vi "Set Next Parameter.vi"(8 "error in (no error)":errorcluster, 10 "first?":bool, 11 "ExperimentService in":refnum<class "ExperimentService.lvclass">) -> (0 "error out":errorcluster, 3 "ExperimentService out":refnum<class "ExperimentService.lvclass">)   [LabVIEW 2014, in "ExperimentService.lvclass"]
uses:
  ExperimentService.lvclass
  ExperimentService.lvclass/ExperimentService.ctl
  Interfaces/Observable Actor/Observable Actor.lvclass
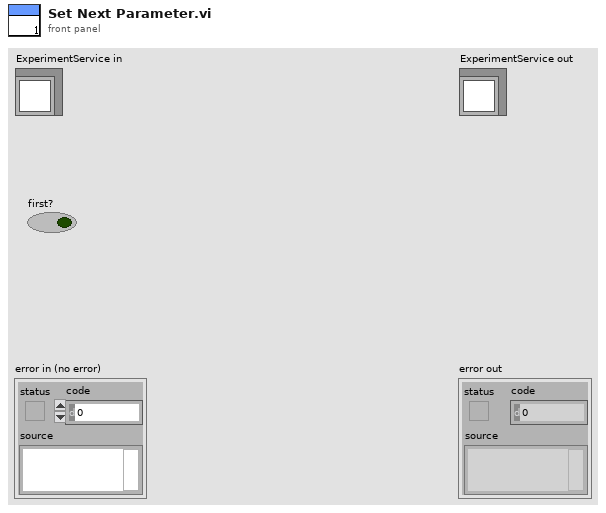
[diagram p1: front panel]
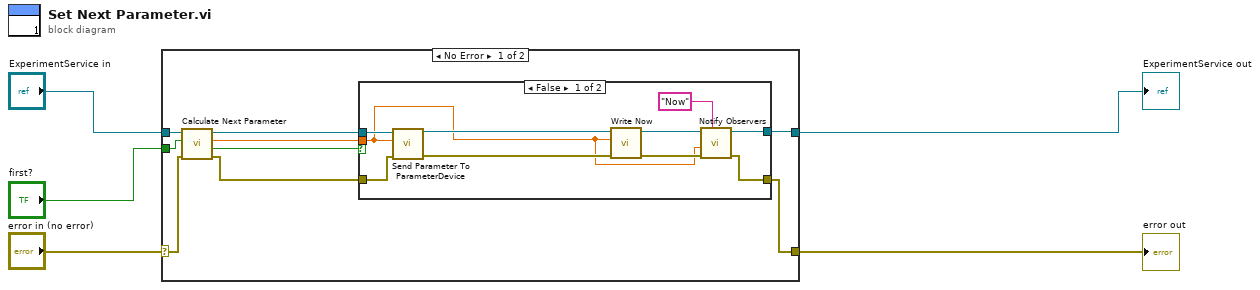
[diagram p0: block diagram]
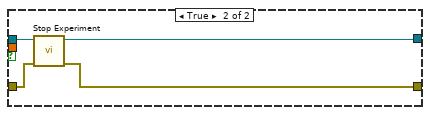
[diagram p2: hidden frame]
diagram:
  n1 = case shown="No Error" "error in (no error)" {
    selector: "error in (no error)" -> [w7 w30]
    tunnel: [w8 w30] -> w1
    tunnel: [w12 w29] -> w2
    tunnel: "ExperimentService in" -> [w14 w29]
    tunnel: "first?" -> [w9 _]
    frame No Error {
      n2 = call-dynamic "Calculate Next Parameter.vi"("error in (no error)"=w7, "first?"=w9, "ExperimentService in"=w14) -> ("error out"=w6:errorcluster, "Stop?"=w10:bool, "Parameter"=w11:dbl, "ExperimentService out"=w13:refnum<class "ExperimentService.lvclass">)  [unwired: 5 in]
      n3 = case shown="False" w10 {
        tunnel: w13 -> [w24 w28]
        tunnel: [w19 w27] -> w12
        tunnel: w11 -> [w15 _]
        tunnel: w6 -> [w22 w26]
        tunnel: [w17 w25] -> w8
        frame False {
          n4 = call-dynamic "Send Parameter To ParameterDevice.vi"("error in (no error)"=w22, "Value"=w15, "ExperimentService in"=w24) -> ("error out"=w21:errorcluster, "ExperimentService out"=w23:refnum<class "ExperimentService.lvclass">)  [unwired: 7 in]
          n5 = call "Write Now.vi"("error in (no error)"=w21, "Now"=w15, "ExperimentService in"=w23) -> ("error out"=w18:errorcluster, "ExperimentService out"=w20:refnum<class "ExperimentService.lvclass">)  [unwired: 7 in]
          n6 = call "Notify Observers.vi"("name"="Now", "error in (no error)"=w18, "value"=w15, "Observable Actor in"=w20) -> ("error out"=w17:errorcluster, "Observable Actor out"=w19:refnum<class "ExperimentService.lvclass">)  [unwired: 6 in]
        }
        frame True {
          n7 = call-dynamic "Stop Experiment.vi"("error in (no error)"=w26, "ExperimentService in"=w28) -> ("error out"=w25:errorcluster, "ExperimentService out"=w27:refnum<class "ExperimentService.lvclass">)  [unwired: 8 in]
        }
      }
    }
    frame Error {
    }
  }
  "error out" <- w1
  "ExperimentService out" <- w2
